vi "Create CLI Report.vi"(8 "error in (no error)":errorcluster, 10 "Results":refnum<class "Report Data.lvclass">[](array[class]), 11 "Report Folder":path) -> (0 "error dub":errorcluster)   [LabVIEW 2019, in "ProjectBuilder.lvlib"]
doc: "Extract a report string for each action and save them to Summary.txt in the report folder (if the report folder exists)."
uses:
  ProjectBuilder.lvlib
  PPL/HDH.ClassLoader.lvlibp
  Class/Data/Report Data/Report Data.lvclass
  <vilib>/Utility/file.llb/Write Delimited Spreadsheet (string).vi
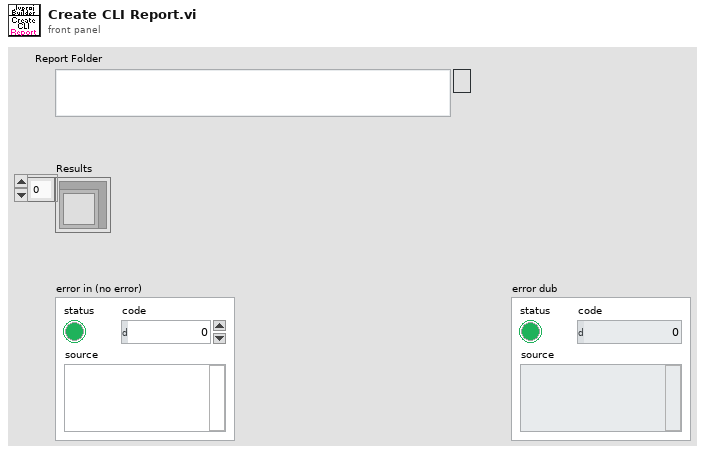
[diagram p1: front panel]
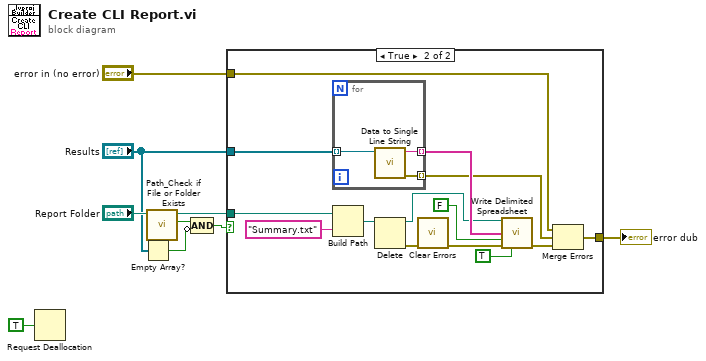
[diagram p0: block diagram]
diagram:
  n1 = Request Deallocation(TRUE ("flag")) -> ()
  n2 = Empty Array?(array="Results") -> (empty?=w9:bool)
  n3 = call "Path_Check if File or Folder Exists.vi"("File or Folder Path in"="Report Folder") -> ("File or Folder Found?"=w6:bool, "File or Folder Path dub"=w5:path)  [unwired: 9 in]
  n4 = Compound Arithmetic op=AND(w6, invert w9) -> (w8:bool)
  n5 = case shown="True" w8 {
    tunnel: w5 -> [_ w23]
    tunnel: [w10 w20] -> w3
    tunnel: "error in (no error)" -> [w10 w12]
    tunnel: "Results" -> [_ w13]
    frame False {
    }
    frame True {
      n6 = for {
        tunnel: [w26] -> w21 mode=indexing
        tunnel: w13 -> [w27] mode=indexing
        tunnel: [w25] -> w11 mode=indexing
        n7 = call "Data to Single Line String.vi"("Report Data in"=w27) -> ("error out"=w25:errorcluster, "Single Line Data"=w26:string)  [unwired: 9 in]
      }
      n8 = Build Path(base path=w23, name or relative path="Summary.txt") -> (appended path=w17:path)
      n9 = Delete(path (use dialog)=w17) -> (deleted path=w16:path, error out=w15:errorcluster)  [unwired: 4 in, 1 out]
      n10 = call <vilib>:"Clear Errors.vi"("error in (no error)"=w15) -> ("error out"=w14:errorcluster)  [unwired: 5 in, 1 out]
      n11 = call-poly <vilib>:"Write Delimited Spreadsheet.vi"("file path (dialog if empty)"=w16, "1D data"=w21, "append to file? (new file:F)"=FALSE, "error in (no error)"=w14, "transpose? (no:F)"=TRUE) -> ("error out"=w19:errorcluster)  [unwired: 9 in, 1 out]
      n12 = Merge Errors(w12, w11, w19) -> (w20:errorcluster)
    }
  }
  "error dub" <- w3
